vi "Fridge Software v2.1.vi"() -> ()   [LabVIEW 2017, in "Fridge Software v2.1.lvlib"]
uses:
  Fridge Software v2.1.lvlib
  <vilib>/Platform/TimedLoop/XDataNode/timing_clust.ctl
  <vilib>/Platform/TimedLoop/XDataNode/nitl_modes.ctl
  <vilib>/Platform/TimedLoop/XDataNode/wakeup.ctl
  <vilib>/Utility/file.llb/Write Delimited Spreadsheet (DBL).vi
  <vilib>/platform/TimedLoop/XDataNode/XDataNode.xnode
  <instrlib>/Lake Shore 372/Lake Shore 372.lvlib
  <instrlib>/Keithley 3706/Keithley 3700 Series.lvlib
  <vilib>/Platform/TimedLoop/XDataNode/XDNodeRunTimeDep.lvlib
panel:
  out "Input Reading Status Query":string
  out "Elapsed time":dbl=500.0 min=50.0 step=100.0
  out "Magnetic Poles \nLive  Voltage":dbl format="%#_5g"
  in  "Measurement\nperiod":i64=500 min=100 step=100
  out "Power Reading":dbl min=0.0 max=0.01 step=1e-05 format="%^.3g"
  out "Sample Reactance":dbl min=0.0 max=63200000.0 step=1e-05 format="%.3g"
  out "Cernox Resistance":dbl min=0.0 max=63200000.0 step=1e-05 format="%.3g"
  in  "R(T,H) tab":enum32{"R(T)", "R(H)"}(tab)
  in  "Clear R(T) graph":bool
  in  "Autoscale R(T)":bool=TRUE caption="Autoscale"
  out "R(T) Graph":cluster{dbl[], dbl[]}(graph)
  in  "Clear H(T) graph":bool
  in  "Autoscale H(T)":bool=TRUE caption="Autoscale"
  out "R(H) Graph":cluster{dbl[], dbl[]}(graph)
  in  "Clear H(t) graph":bool
  in  "Clear T(t) graph":bool
  in  "Clear R(t) graph":bool
  out "Sample Resistance":dbl min=0.0 max=63200000.0 step=1e-05 format="%^.5g"
  out "Cernox Temperature":dbl min=0.0 max=1000.0 step=1e-05 format="%.4f"
  in  "Autoscale H(t)":bool=TRUE caption="Autoscale"
  in  "Autoscale T(t)":bool=TRUE caption="Autoscale"
  in  "Autoscale R(t)":bool=TRUE caption="Autoscale"
  out "H(t) Graph 4":cluster{dbl[], dbl[]}(graph)
  out "T(t) Graph 3":cluster{dbl[], dbl[]}(graph)
  out "R(t) Graph":cluster{dbl[], dbl[]}(graph)
  in  "Measurement":T1(tab)
  in  "Hall probe/Aux":bool
  in  "Lakeshore port":refnum<visa-resource-name>="COM6"
  in  "Cernox Channel":u16(ring)=17 caption="Cernox" items=["1"=1, "2"=2, "3"=3, "4"=4, "5"=5, "6"=6, "7"=7, "8"=8, "9"=9, "10"=10, "11"=11, "12"=12, "13"=13, "14"=14, "15"=15, "16"=16, "A"=17]
  in  "Sample Channel":u16(ring)=1 caption="Sample" items=["1"=1, "2"=2, "3"=3, "4"=4, "5"=5, "6"=6, "7"=7, "8"=8, "9"=9, "10"=10, "11"=11, "12"=12, "13"=13, "14"=14, "15"=15, "16"=16, "A (Control Input)"=17]
  in  "Switchboard port":refnum<visa-resource-name>="USB0::0x05E6::0x3706::04089883::INSTR"
  in  "Arduino port \n(for magnetic poles)":refnum<visa-resource-name>="COM3"
  out "Lakeshore Error":errorcluster
  in  "Update":bool
  out "Excitation  Ind":bool=TRUE
  out "Excitation Mode Ind":u16(ring)=1 items=["Voltage", "Current"]
  out "Excitation Range Ind":u16(ring)=19 items=["31.6 mA"=22, "10.0 mA"=21, "3.16 mA"=20, "1.00 mA"=19, "316 uA"=18, "100 uA"=17, "31.6 uA"=16, "10.0 uA"=15, "3.16 uA"=14, "1.00 uA"=13, "632 mV / 316 nA"=12, "200 mV / 100 nA"=11, "63.2 mV / 31.6 nA"=10, "20.0 mV / 10.0 nA"=9, "6.32 mV / 3.16 nA"=8, "2.00 mV / 1.00 nA"=7, "632 uV / 316 pA"=6, "200 uV / 100 pA"=5, "63.2 uV / 31.6 pA"=4, "20.0 uV / 10.0 pA"=3, "6.32 uV / 3.16 pA"=2, "2.00 uV / 1.00 pA"=1]
  out "Autorange Ind":u16(ring) items=["Autorange off", "Autorange Current", "ROX 102B Autorange"]
  out "Resistance Range Ind":u16(ring)=8 items=["63.2 MOhm"=22, "20.0 MOhm"=21, "6.32 MOhm"=20, "2.00 MOhm"=19, "632 kOhm"=18, "200 kOhm"=17, "63.2 kOhm"=16, "20.0 kOhm"=15, "6.32 kOhm"=14, "2.00 kOhm"=13, "632 Ohm"=12, "200 Ohm"=11, "63.2 Ohm"=10, "20.0 Ohm"=9, "6.32 Ohm"=8, "2.00 Ohm"=7, "632 mOhm"=6, "200 mOhm"=5, "63.2 mOhm"=4, "20.0 mOhm"=3, "6.32 mOhm"=2, "2.00 mOhm"=1]
  out "Preferred Units Ind":u16(ring)=2 items=["Kelvin"=1, "Ohms"=2]
  out "Temperature Limit Ind":dbl min=0.0 max=2999.0 step=1.0
  in  "Excitation Mode":u16(ring)=1 items=["Voltage", "Current"]
  in  "Excitation Range":u16(ring)=19 items=["31.6 mA"=22, "10.0 mA"=21, "3.16 mA"=20, "1.00 mA"=19, "316 uA"=18, "100 uA"=17, "31.6 uA"=16, "10.0 uA"=15, "3.16 uA"=14, "1.00 uA"=13, "632 mV / 316 nA"=12, "200 mV / 100 nA"=11, "63.2 mV / 31.6 nA"=10, "20.0 mV / 10.0 nA"=9, "6.32 mV / 3.16 nA"=8, "2.00 mV / 1.00 nA"=7, "632 uV / 316 pA"=6, "200 uV / 100 pA"=5, "63.2 uV / 31.6 pA"=4, "20.0 uV / 10.0 pA"=3, "6.32 uV / 3.16 pA"=2, "2.00 uV / 1.00 pA"=1]
  in  "Autorange (0: Autorange off)":u16(ring) items=["Autorange off", "Autorange Current", "ROX 102B Autorange"]
  in  "Resistance Range":u16(ring)=8 items=["63.2 MOhm"=22, "20.0 MOhm"=21, "6.32 MOhm"=20, "2.00 MOhm"=19, "632 kOhm"=18, "200 kOhm"=17, "63.2 kOhm"=16, "20.0 kOhm"=15, "6.32 kOhm"=14, "2.00 kOhm"=13, "632 Ohm"=12, "200 Ohm"=11, "63.2 Ohm"=10, "20.0 Ohm"=9, "6.32 Ohm"=8, "2.00 Ohm"=7, "632 mOhm"=6, "200 mOhm"=5, "63.2 mOhm"=4, "20.0 mOhm"=3, "6.32 mOhm"=2, "2.00 mOhm"=1]
  in  "Preferred Units (2: Ohms)":u16(ring)=2 items=["Kelvin"=1, "Ohms"=2]
  in  "Temperature Limit (0 Kelvin)":dbl min=0.0 max=2999.0 step=1.0
  in  "Excitation  (T: On)":bool=TRUE caption="On\n\nOff"
  in  "Grab settings":bool
  out "Heater Output Ind":dbl
  in  "Heater Setpoint":dbl
  out "Heater Setpoint Ind":dbl
  in  "Grab Heater settings":bool
  in  "Update Heater Settings":bool
  in  "Excitation  (T: On) 2":bool=TRUE caption="On\n\nOff"
  out "Excitation  Ind 2":bool=TRUE
  out "Heater Output Ind 2":dbl
  in  "I+":i32 min=0 max=24 step=1
  in  "I-":i32 min=0 max=24 step=1
  in  "V+":i32 min=0 max=24 step=1
  in  "V-":i32 min=0 max=24 step=1
  in  "Close pins (safe)":bool caption="Close I-V pins -> Lift ground -> Lift common -> Current on"
  in  "Lift pins (safe)":bool caption="Current off -> Common closed -> Ground -> Lift I-V pins"
  in  "Channel Open/Close Array":string
  in  "Open":bool
  in  "Close":bool
  in  "Open All IV":bool
  out "Closed Channels":string
  out "Ground closed":bool
  out "Common rail \nclosed":bool
  out "Common-ground \nlink closed":bool
  in  "Append file":bool
  in  "File path":path
  in  "Save Data":bool
  in  "error in":errorcluster
  in  "Aux max voltage (mV)":dbl
  in  "Aux Field Range (Oe)":dbl
  in  "Stop":bool
  # "Created by Daniel Bromley & Alex Wright, IPF Ltd 2021"
  # "s"
  # "V"
  # "ms"
  # "W"
  # "jW"
  # "W"
  # "W"
  # "K"
  # "Lakeshore - Measurement"
  # "Channels:"
  # "Keithley - Switchboard"
  # "Hall probe"
  # "Aux"
  # "Excitation Mode"
  # "Excitation Range"
  # "Autorange"
  # "Resistance Range"
  # "Preferred Units"
  # "Temperature Limit"
  # "Excitation"
  # "Heater Serpoint (K)"
  # "Heater output"
  # "Heater On"
  # "IV pins"
  # "Array"
  # "Set Filename and Path"
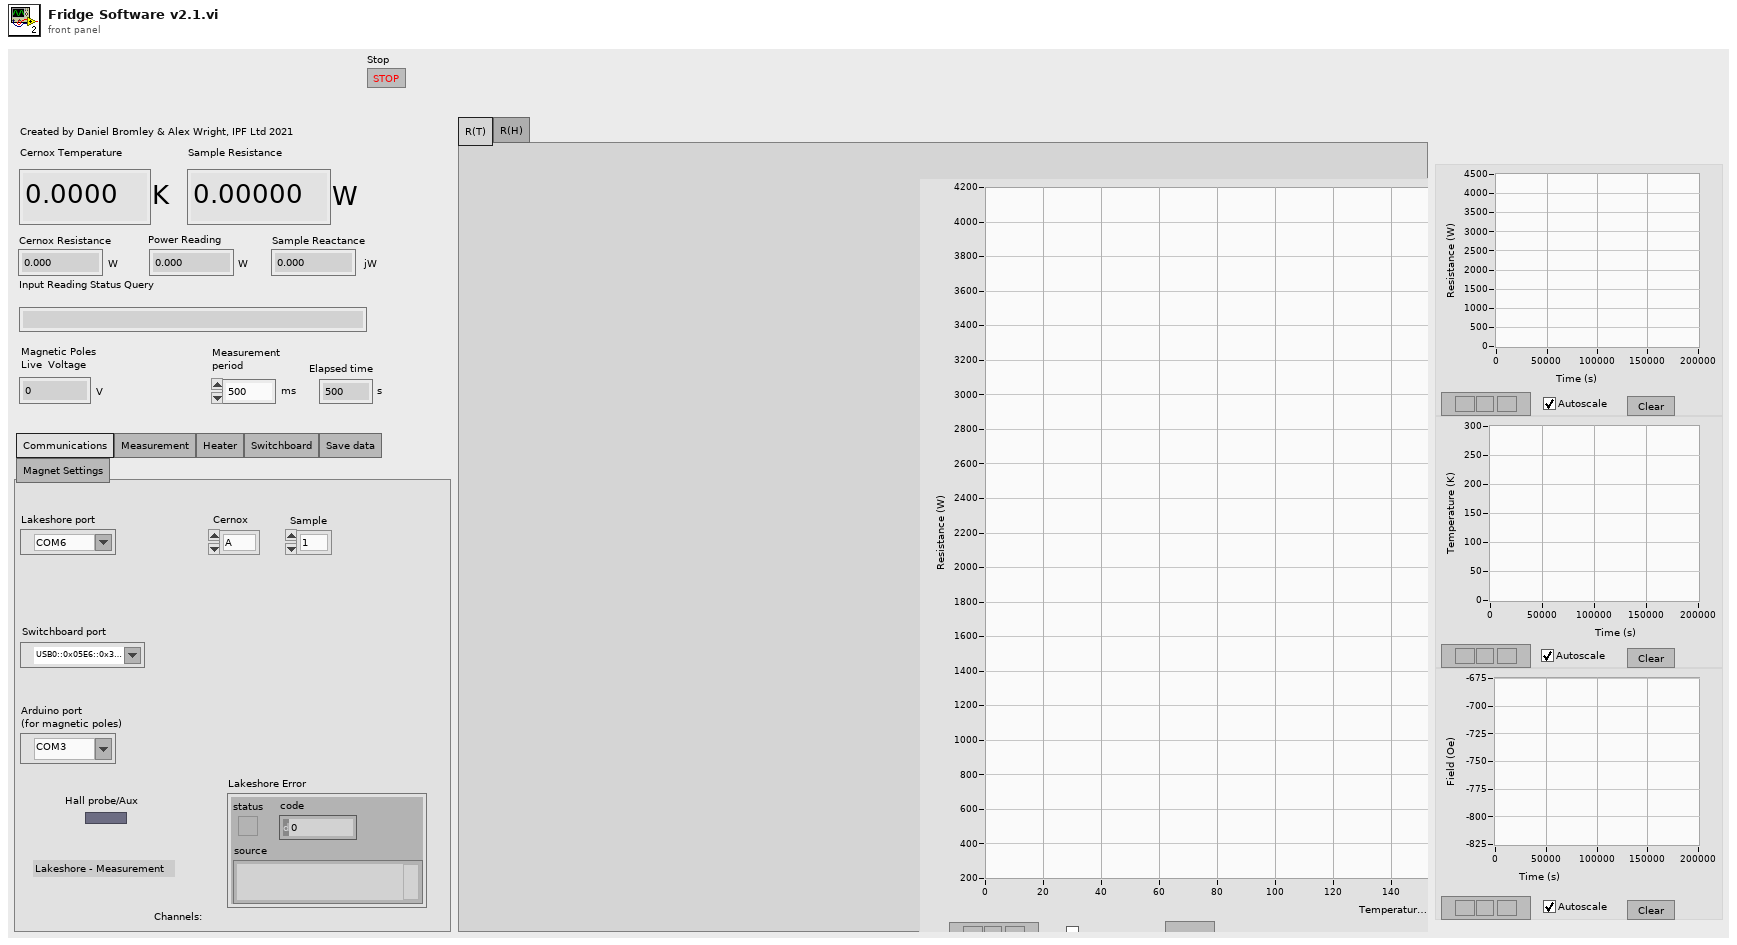
[diagram p1: front panel]
types:
  T1 = enum32{"Communications", "Measurement", "Heater", "Switchboard", "Save data", "Magnet Settings"}
  T2 = typedef "XDNodeRunTimeDep.lvlib/timing_clust.ctl" = cluster{"Expected End [f-1]":u64, "Actual End [f-1]":u64, "Finished Late? [f-1]":bool, "Expected End [i-1]":u64, "Actual End [i-1]":u64, "Finished Late? [i-1]":bool, "Expected Start [i]":u64, "Actual Start [i]":u64, "Expected Start [f]":u64, "Actual Start [f]":u64, "Source Name":string, "Structure Name":string, "Period":i64, "Deadline":i64, "Offset":i64, "Start":i64, "Priority":i32, "Timeout":i32, "Mode":T3, "Wakeup Reason":T4, "Error":errorcluster, "Source Type":string, "Secondary Source Type":string, "Global End Time":u64, "Global Start Time":u64, "Frame Duration":u64, "Iteration Duration":u64, "Assigned CPU":i32, "I/O Scan Engine Mode":u32}
  T3 = typedef "XDNodeRunTimeDep.lvlib/nitl_modes.ctl" = enum32{"No Change", "Process missed periods, maintain original phase", "Discard missed periods, maintain original phase", "Process missed periods, ignore original phase", "Discard missed periods, ignore original phase"}
  T4 = typedef "XDNodeRunTimeDep.lvlib/wakeup.ctl" = enum32{"Normal", "Aborted", "Asynchronous wakeup", "Timing source error", "Timed loop error", "Timeout"}
  T5 = typedef "eventsource.ctl" = u32
  T6 = typedef "lveventtype.ctl" = enum32{"Null", "Timeout", "Annotation Menu Selection", "Annotation Menu Selection?", "App Instance Close", "App Instance Close?", "Autoscale Range Change", "Bookmark Info Change", "Cell Edit", "Cell Edit?", "Cursor Grab", "Cursor Grab?", "Cursor Menu Selection", "Cursor Menu Selection?", "Cursor Move", "Cursor Release", "Data Change", "Direction Change", "Display State Change", "Drag Ended", "Drag Enter", "Drag Leave", "Drag Over", "Drag Source Update", "Drag Starting", "Drag Starting?", "Drop", "Exec State Change", "Key Down", "Key Down?", "Key Repeat", "Key Repeat?", "Key Up", "Listbox Double Click", "Menu Activation?", "Menu Selection (App)", "Menu Selection? (App)", "Menu Selection (User)", "Mouse Down", "Mouse Down?", "Mouse Enter", "Mouse Leave", "Mouse Move", "Mouse Up", "Mouse Wheel", "NI Security User Change (App)", "Pane Size", "Panel Close", "Panel Close?", "Panel Resize", "Plot Attribute Change", "Scale Range Change", "Shortcut Menu Activation?", "Shortcut Menu Selection (App)", "Shortcut Menu Selection? (App)", "Shortcut Menu Selection (User)", "Tree Double Click", "Tree Drag", "Tree Drag?", "Tree Drop", "Tree Drop?", "Tree Item Close", "Tree Item Close?", "Tree Item Open", "Tree Item Open?", "User Event", "Value Change"}
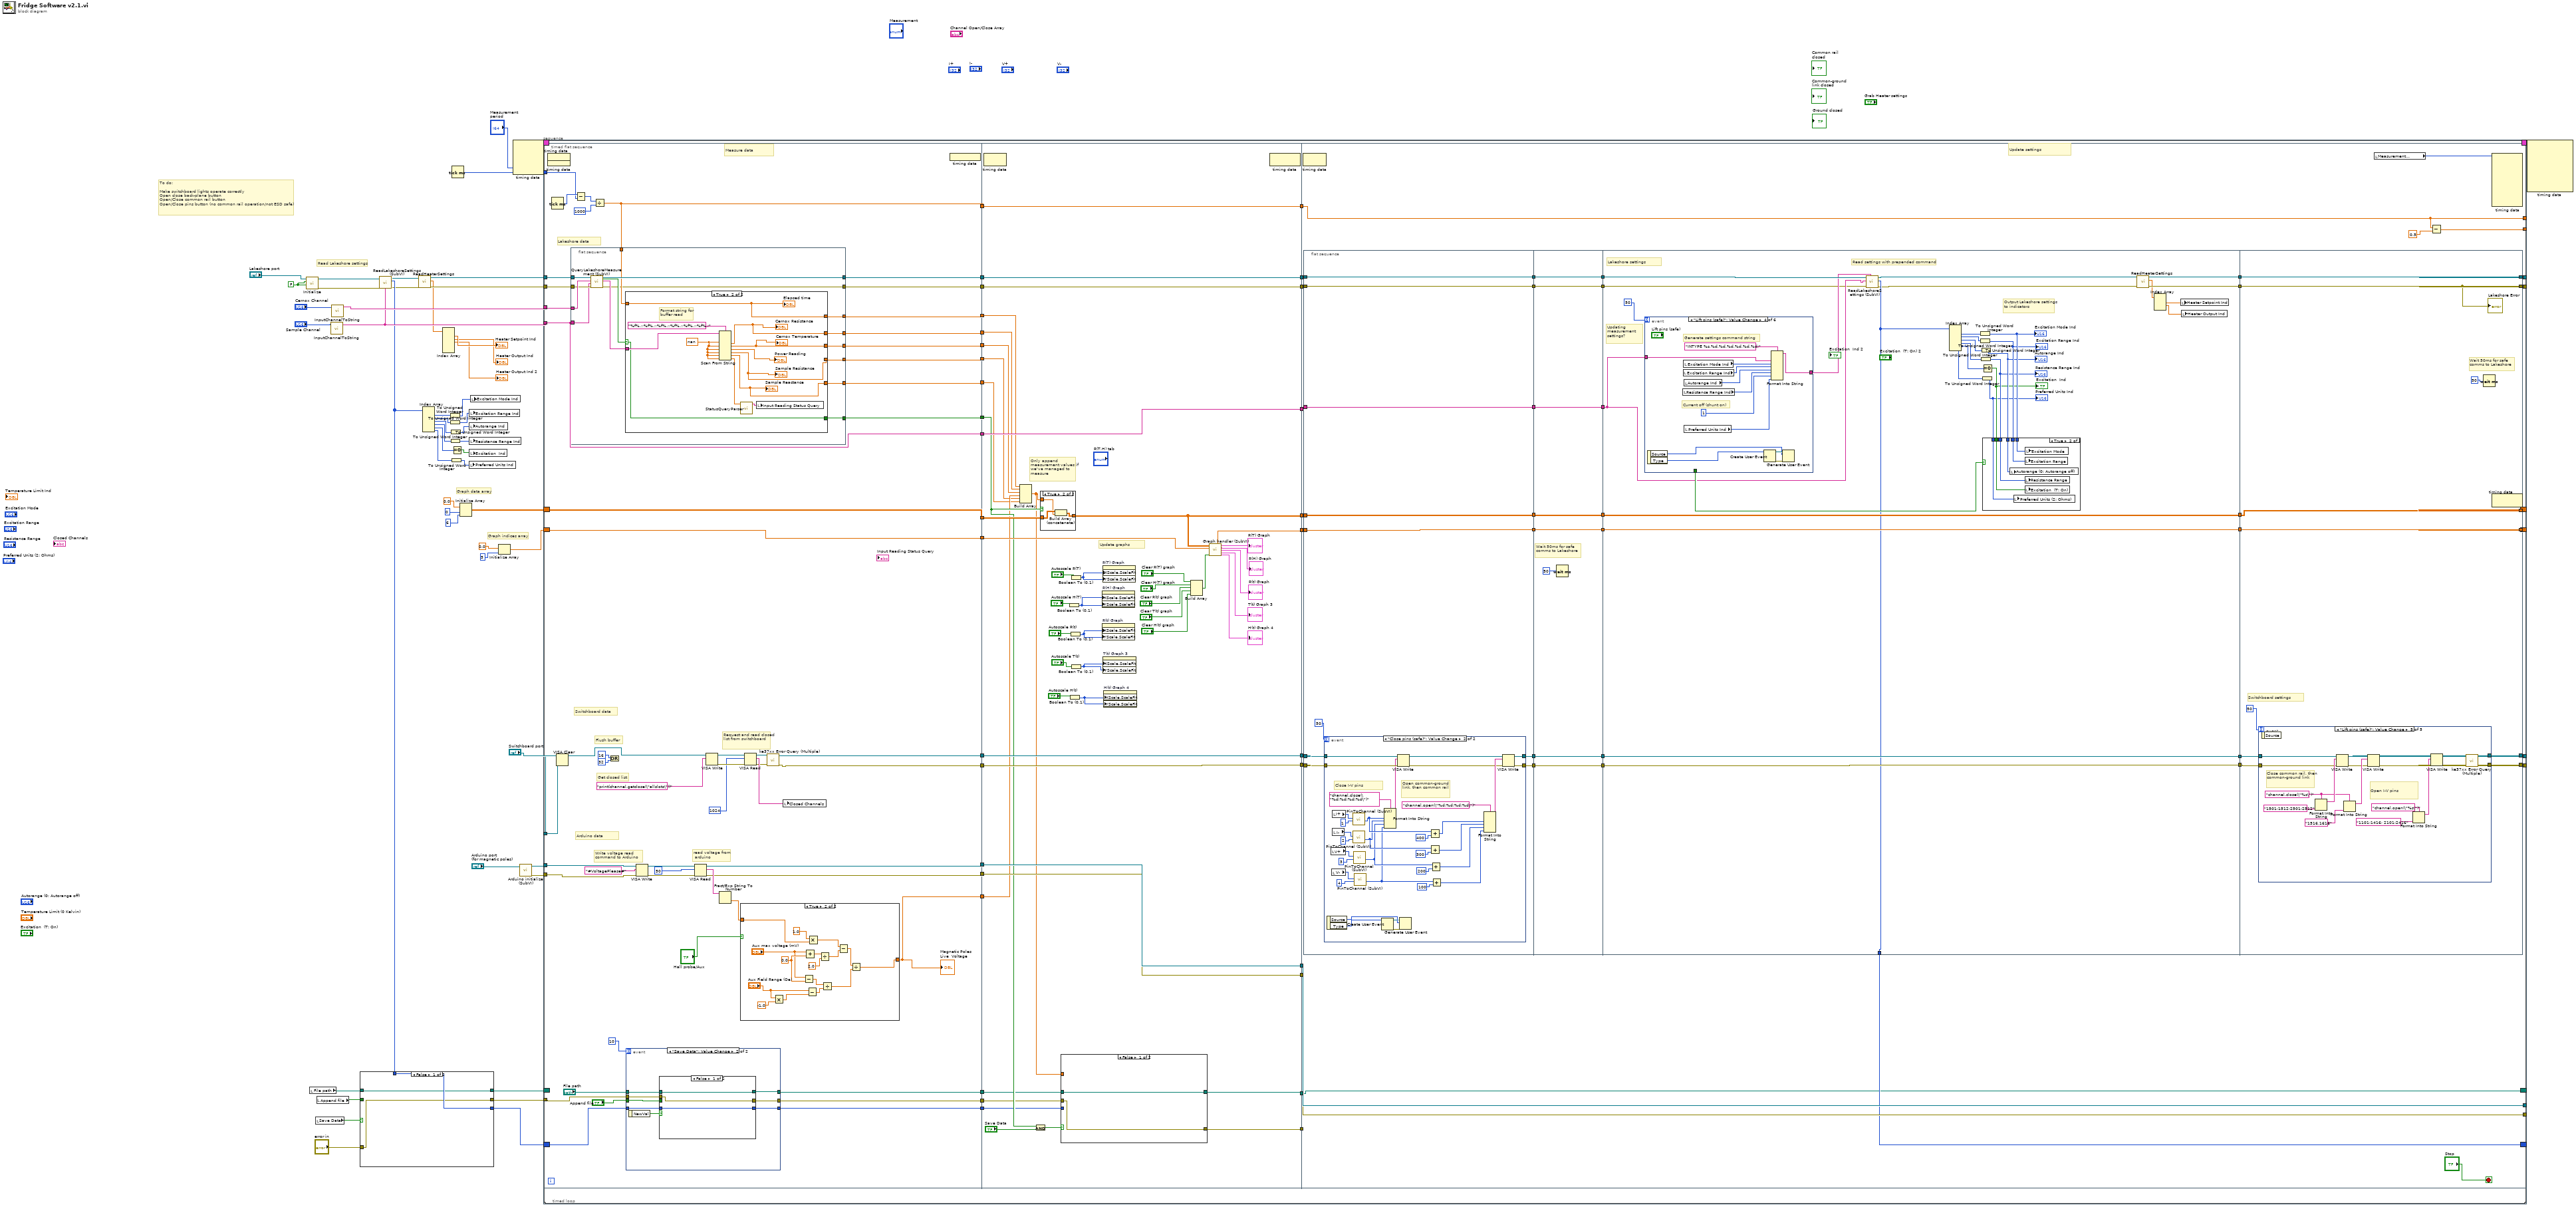
[diagram p0: block diagram]
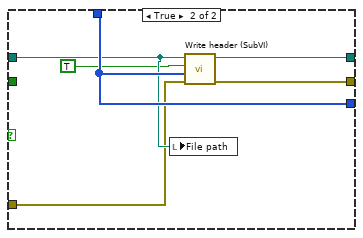
[diagram p2: hidden frame]
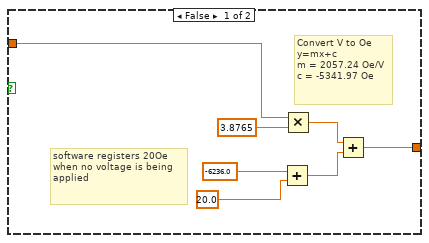
[diagram p3: hidden frame]
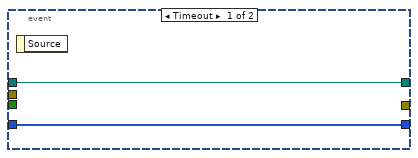
[diagram p4: hidden frame]
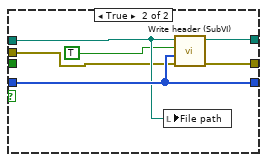
[diagram p5: hidden frame]
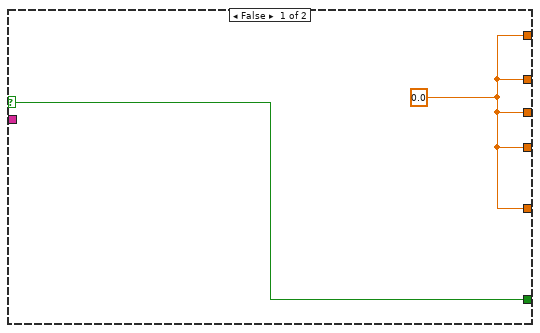
[diagram p6: hidden frame]
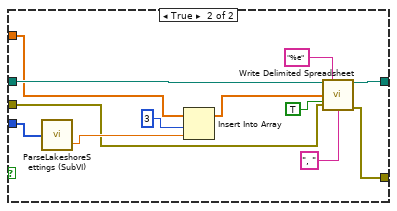
[diagram p7: hidden frame]
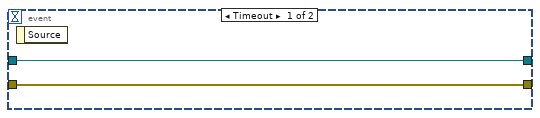
[diagram p9: hidden frame]
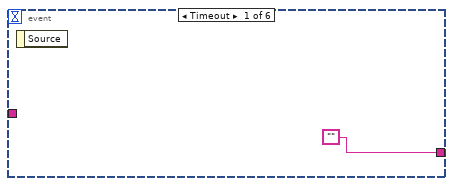
[diagram p10: hidden frame]
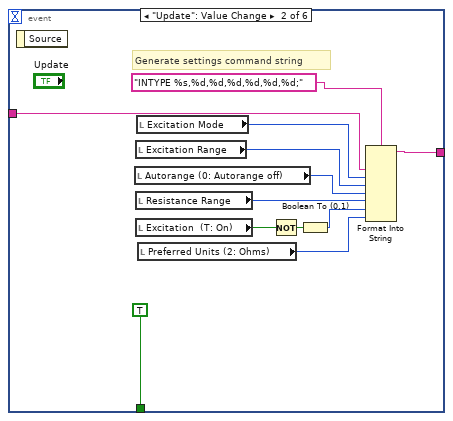
[diagram p11: hidden frame]
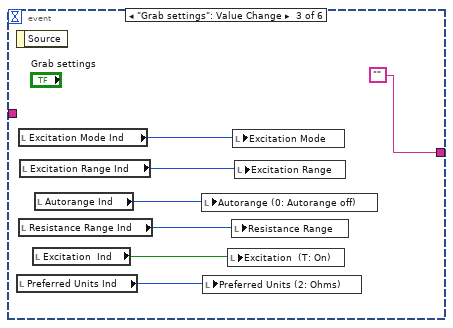
[diagram p12: hidden frame]
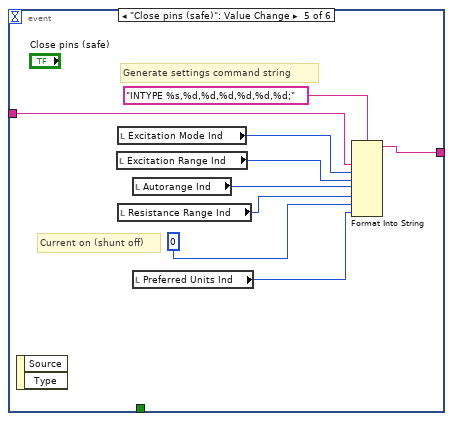
[diagram p13: hidden frame]
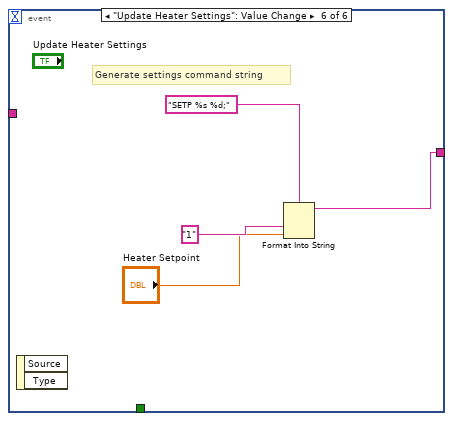
[diagram p14: hidden frame]
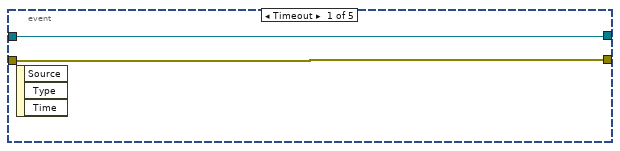
[diagram p16: hidden frame]
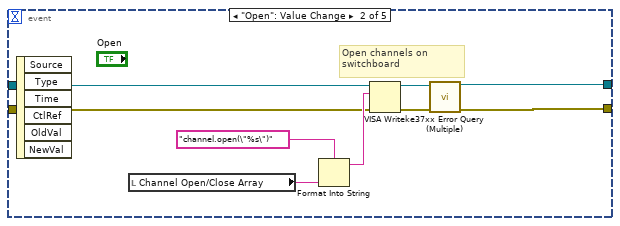
[diagram p17: hidden frame]
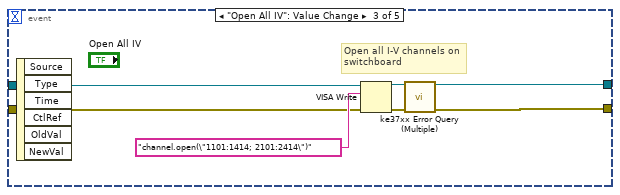
[diagram p18: hidden frame]
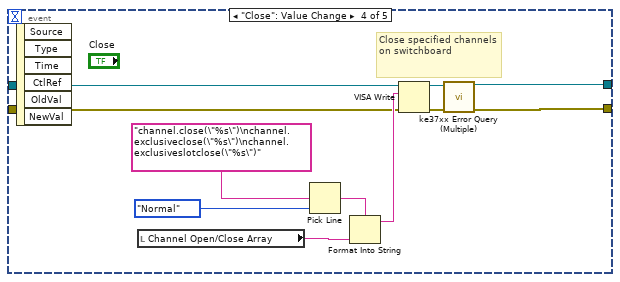
[diagram p19: hidden frame]
diagram:
  w12 = FALSE
  # "To do:\n\nMake switchboard lights operate correctly\nOpen close back-plane button\nOpen/Close common rail button\nOpen/Close pins button (no common rail operation/not ESD safe)"
  # "Read Lakeshore settings"
  # "Graph indices array"
  # "Graph data array"
  n1 = call <instrlib>:"Initialize.vi"("Reset (True)"=w12, "ID Query (True)"=w12, "VISA resource name"="Lakeshore port") -> ("error out"=w11:errorcluster, "VISA resource name out"=w32:refnum<visa-resource-name>)  [unwired: 7 in]
  n2 = local read "File path"() -> (w13:path)
  n3 = local read "Save Data"() -> (w24:bool)
  n4 = local read "Append file"() -> (w23:bool)
  n5 = call <instrlib>:"InputChannelToString.vi"("Channel (1)"="Sample Channel") -> ("Channel Str"=w28:string)  [unwired: 10 in]
  n6 = call <instrlib>:"InputChannelToString.vi"("Channel (1)"="Cernox Channel") -> ("Channel Str"=w30:string)  [unwired: 10 in]
  n7 = call "ReadLakeshoreSettings (SubVI).vi"("error in (no error)"=w11, "Channel Str"=w28, "Lakeshore port"=w32) -> ("error out"=w8:errorcluster, "Settings array out"=w22:i32[], "VISA Refnum out"=w10:refnum<visa-resource-name>)  [unwired: 4 in]
  n8 = case shown="False" w24 {
    tunnel: w23 -> [_ _]
    tunnel: w22 -> [w55 w61]
    tunnel: [w55 w61] -> w21
    tunnel: [w54 w60] -> w14
    tunnel: w13 -> [w54 w59]
    tunnel: [w53 w57] -> w2
    tunnel: "error in" -> [w53 w56]
    frame False {
    }
    frame True {
      n9 = local write "File path"(w59) -> ()
      n10 = call "Write header (SubVI).vi"("error in"=w56, "Settings array in"=w61, "Append? Out"=TRUE, "Path in"=w59) -> ("error out"=w57:errorcluster, "Path out"=w60:path)  [unwired: 6 in]
    }
  }
  n11 = call "ReadHeaterSettings.vi"("error in (no error)"=w8, "VISA Refnum in"=w10) -> ("error out"=w7:errorcluster, "Settings array out"=w6:dbl[], "VISA Refnum out"=w9:refnum<visa-resource-name>)  [unwired: 7 in]
  n12 = Index Array(array=w22) -> (element #1=w38:i32, element #2=w37:i32, element #3=w36:i32, element #4=w35:i32, element #5=w34:i32, element #6=w33:i32)  [unwired: 6 in]
  n13 = Index Array(array=w6) -> (element #1=→"Heater Setpoint Ind":dbl, element #2=→"Heater Output Ind":dbl, element #3=→"Heater Output Ind 2":dbl)  [unwired: 6 in, 3 out]
  n14 = To Unsigned Word Integer(number=w38) -> (unsigned 16bit integer=w20:u16)
  n15 = To Unsigned Word Integer(number=w37) -> (unsigned 16bit integer=w19:u16)
  n16 = To Unsigned Word Integer(number=w35) -> (unsigned 16bit integer=w17:u16)
  n17 = To Unsigned Word Integer(number=w36) -> (unsigned 16bit integer=w18:u16)
  n18 = To Unsigned Word Integer(number=w33) -> (unsigned 16bit integer=w15:u16)
  n19 = Equal To 0?(x=w34) -> (x = 0?=w16:bool)
  n20 = Tick Count (ms)() -> (millisecond timer value=w51:u32)
  n21 = Initialize Array(0.0, 0, 6) -> (w42:dbl[][])
  n22 = local write "Preferred Units Ind"(w15) -> ()
  n23 = local write "Excitation Range Ind"(w19) -> ()
  n24 = local write "Autorange Ind"(w18) -> ()
  n25 = local write "Resistance Range Ind"(w17) -> ()
  n26 = local write "Excitation  Ind"(w16) -> ()
  n27 = local write "Excitation Mode Ind"(w20) -> ()
  n28 = Initialize Array(0.0, 5) -> (w39:dbl[])
  n29 = node-c288("Measurement\nperiod") -> (w50:T2)  [unwired: 3 in]
  n30 = call "Arduino initialize (SubVI).vi"("VISA Refnum in"="Arduino port \n(for magnetic poles)") -> ("error out"=w25:errorcluster, "VISA Refnum out"=w26:refnum<visa-resource-name>)  [unwired: 9 in]
  n31 = VISA Clear(VISA resource name="Switchboard port") -> (VISA resource name out=w46:refnum<visa-resource-name>)  [unwired: 1 in, 1 out]
  n32 = timed-loop {
    timing: w50 -> [_]
    timing-out: [_] -> w49
    tunnel: w30 -> [w86]
    tunnel: w28 -> [w85]
    tunnel: w7 -> [w84]
    tunnel: w9 -> [w83]
    tunnel: w26 -> [w82]
    tunnel: w25 -> [w81]
    tunnel: [w80] -> _
    tunnel: [w79] -> _
    tunnel: [w78] -> _
    tunnel: [w77] -> _
    tunnel: w46 -> [w76]
    tunnel: w51 -> [w75]
    tunnel: [w74] -> _
    tunnel: [w73] -> _
    shift-right: [w72] -> _
    shift-left: w42 -> [w71]
    shift-right: [w70] -> _
    shift-left: w39 -> [w69]
    tunnel: [w68] -> _
    tunnel: [w67] -> _
    shift-right: [w66] -> _
    shift-left: w21 -> [w65]
    shift-right: [w64] -> _
    shift-left: w14 -> [w63]
    tunnel: w2 -> [w62]
    stop <- "Stop" stop-if-true
    n33 = timed-sequence {
      timing: _ -> [_]
      timing-out: _ -> [_]
      tunnel: w86 -> [w140]
      tunnel: w85 -> [w143]
      tunnel: w84 -> [w142]
      tunnel: w83 -> [w141]
      tunnel: w82 -> [w135]
      tunnel: w81 -> [w134]
      tunnel: [w139] -> w80
      tunnel: [w138] -> w79
      tunnel: [w137] -> w78
      tunnel: [w136] -> w77
      tunnel: w76 -> [w133]
      tunnel: w75 -> [w132]
      tunnel: [w131] -> w74
      tunnel: [w130] -> w73
      tunnel: [w129] -> w72
      tunnel: w71 -> [w128]
      tunnel: [w102] -> w70
      tunnel: w69 -> [w100]
      tunnel: [w98] -> w68
      tunnel: [w97] -> w67
      tunnel: [w96] -> w66
      tunnel: w65 -> [w95]
      tunnel: [w94] -> w64
      tunnel: w63 -> [w93]
      tunnel: w62 -> [w89]
      n34 = timed-flat-sequence {
        tunnel: w143 -> [w192]
        tunnel: [w194] -> w127
        tunnel: [w193] -> w125
        tunnel: [w192] -> w123
        tunnel: w142 -> [w191]
        tunnel: w141 -> [w190]
        tunnel: w140 -> [w189]
        tunnel: [w185] -> w121
        tunnel: [w184] -> w119
        tunnel: w135 -> [w170]
        tunnel: w134 -> [w169]
        tunnel: w133 -> [w171]
        tunnel: [w156] -> w117
        tunnel: [w155] -> w115
        tunnel: w132 -> [w167]
        tunnel: [w158] -> w113
        tunnel: w128 -> [w166]
        tunnel: [w166] -> w111
        tunnel: [w165] -> w110
        tunnel: [w164] -> w109
        tunnel: [w163] -> w108
        tunnel: [w162] -> w107
        tunnel: [w161] -> w106
        tunnel: [w146] -> w105
        tunnel: [w160] -> w103
        tunnel: [w159] -> w101
        tunnel: w100 -> [w159]
        tunnel: w95 -> [w154]
        tunnel: w93 -> [_]
        tunnel: [w150] -> w92
        tunnel: [w149] -> w90
        tunnel: w89 -> [w145]
        tunnel: [w144] -> w88
        tunnel: w127 -> [w315]
        tunnel: [w315] -> w126
        tunnel: w125 -> [w314]
        tunnel: [w314] -> w124
        tunnel: w123 -> [w313]
        tunnel: [w313] -> w122
        tunnel: w121 -> [w312]
        tunnel: [w312] -> w120
        tunnel: w119 -> [w311]
        tunnel: [w311] -> w118
        tunnel: w117 -> [w310]
        tunnel: [w310] -> w116
        tunnel: w115 -> [w309]
        tunnel: [w309] -> w114
        tunnel: w113 -> [w308]
        tunnel: [w308] -> w112
        tunnel: w111 -> [w307]
        tunnel: w110 -> [w306]
        tunnel: w109 -> [w305]
        tunnel: w108 -> [w304]
        tunnel: w107 -> [w271]
        tunnel: w106 -> [w270]
        tunnel: w105 -> [w272]
        tunnel: [w288] -> w104
        tunnel: w103 -> [w278]
        tunnel: w101 -> [w287]
        tunnel: [w285] -> w99
        tunnel: w92 -> [w275]
        tunnel: [w274] -> w91
        tunnel: w90 -> [w273]
        tunnel: w88 -> [w269]
        tunnel: [w268] -> w87
        tunnel: w126 -> [w377]
        tunnel: w124 -> [w376]
        tunnel: w122 -> [w375]
        tunnel: [w374] -> w139
        tunnel: [w373] -> w138
        tunnel: w120 -> [w372]
        tunnel: w118 -> [w371]
        tunnel: [w372] -> w137
        tunnel: [w371] -> w136
        tunnel: w116 -> [w366]
        tunnel: w114 -> [w365]
        tunnel: w112 -> [w339]
        tunnel: [w368] -> w131
        tunnel: [w367] -> w130
        tunnel: [w346] -> w129
        tunnel: w104 -> [w348]
        tunnel: [w341] -> w102
        tunnel: w99 -> [w344]
        tunnel: [w339] -> w98
        tunnel: [w338] -> w97
        tunnel: [w337] -> w96
        tunnel: [w336] -> w94
        tunnel: w91 -> [w336]
        tunnel: w87 -> [_]
        frame #0 {
          # "Request and read closed list from switchboard"
          # "Get closed list"
          # "Flush buffer"
          # "Switchboard data"
          # "Arduino data"
          # "Lakeshore data"
          # "read voltage from\n arduino"
          # "Write voltage read command to Arduino"
          # "Measure data"
          n35 = node-c288() -> ()  [unwired: 1 in]
          n36 = Tick Count (ms)() -> (millisecond timer value=w168:u32)
          n37 = flat-sequence {
            tunnel: w192 -> [w245]
            tunnel: w191 -> [w249]
            tunnel: w190 -> [w248]
            tunnel: w189 -> [w250]
            tunnel: [w251] -> w194
            tunnel: [w237] -> w193
            tunnel: w158 -> [w244]
            tunnel: [w243] -> w165
            tunnel: [w242] -> w164
            tunnel: [w241] -> w163
            tunnel: [w240] -> w162
            tunnel: [w239] -> w161
            tunnel: [w238] -> w160
            frame #0 {
              n38 = call "QueryLakeshoreMeasurement (SubVI).vi"("error in (no error)"=w249, "Sample Channel Str"=w245, "Cernox channel string"=w250, "VISA Refnum in"=w248) -> ("error out"=w237:errorcluster, "Read output"=w247:string, "VISA Refnum out"=w251:refnum<visa-resource-name>, "Boolean"=w246:bool)  [unwired: 4 in]
              n39 = case shown="True" w246 {
                selector: w246 -> [w252 w262]
                tunnel: w247 -> [_ w264]
                tunnel: w244 -> [_ w259]
                tunnel: [w253 w259] -> w243
                tunnel: [w253 w257] -> w242
                tunnel: [w253 w256] -> w241
                tunnel: [w253 w254] -> w240
                tunnel: [w253 w258] -> w239
                tunnel: [w252 w262] -> w238
                frame False {
                  w253 = 0.0
                }
                frame True {
                  w263 = nan
                  # "Format string for buffer read"
                  n40 = Scan From String(format string="%f%.;;%f%.;;%f%.;;%f%.;;%f%.;;%f%.;", input string=w264, default 1=w263, default 2=w263, default 3=w263, default 4=w263, default 5=w263, default 6=w263) -> (output 1=w257:dbl, output 2=w256:dbl, output 3=→"Power Reading":dbl, output 4=w254:dbl, output 5=w258:dbl, output 6=w261:dbl)  [unwired: 2 in, 3 out]
                  "Sample Reactance" <- w258
                  "Cernox Resistance" <- w257
                  "Cernox Temperature" <- w256
                  "Sample Resistance" <- w254
                  n41 = call "StatusQueryParser.vi"("Numeric"=w261) -> ("String"=w260:string)  [unwired: 10 in]
                  n42 = local write "Input Reading Status Query"(w260) -> ()
                  "Elapsed time" <- w259
                }
              }
            }
          }
          n43 = Subtract(x=w168, y=w167) -> (x-y=w174:u32)
          n44 = Divide(x=w174, y=1000) -> (x/y=w158:dbl)
          n45 = Or(x=16, y=32) -> ()  [unwired: 1 out]
          n46 = event shown="[1] \"Save Data\": Value Change" {
            selector: _ -> [_ _]
            dyn-events: _ -> [_ _]
            timeout: 10 -> [_ _]
            tunnel: w154 -> [w218 w226]
            tunnel: "Append file" -> [_ w225]
            tunnel: "File path" -> [w219 w224]
            tunnel: [w219 w223] -> w150
            tunnel: [w218 w222] -> w149
            tunnel: w145 -> [_ w221]
            tunnel: [_ w220] -> w144
            event Timeout {
              n47 = event-data() -> ()  [unwired: 1 in, 1 out]
            }
            event "Save Data": Value Change {
              n48 = event-data() -> ("NewVal"=w227:bool)  [unwired: 1 in]
              n49 = case shown="False" w227 {
                tunnel: w226 -> [w229 w235]
                tunnel: w225 -> [_ _]
                tunnel: w224 -> [w230 w234]
                tunnel: [w230 w236] -> w223
                tunnel: [w229 w235] -> w222
                tunnel: w221 -> [w228 w232]
                tunnel: [w228 w231] -> w220
                frame False {
                }
                frame True {
                  n50 = local write "File path"(w234) -> ()
                  n51 = call "Write header (SubVI).vi"("error in"=w232, "Settings array in"=w235, "Append? Out"=TRUE, "Path in"=w234) -> ("error out"=w231:errorcluster, "Path out"=w236:path)  [unwired: 6 in]
                }
              }
            }
          }
          n52 = VISA Write(VISA resource name=w170, write buffer="#VoltagePlease#" ("Send to Arduino"), error in (no error)=w169) -> (VISA resource name out=w186:refnum<visa-resource-name>, error out=w183:errorcluster)  [unwired: 1 out]
          n53 = VISA Read(VISA resource name=w186, byte count=u32 50 ("milliseconds to wait"), error in (no error)=w183) -> (VISA resource name out=w185:refnum<visa-resource-name>, read buffer=w188:string, error out=w184:errorcluster)  [unwired: 1 out]
          n54 = VISA Write(VISA resource name=w171, write buffer="print(channel.getclose(\"allslots\"))") -> (VISA resource name out=w180:refnum<visa-resource-name>, error out=w179:errorcluster)  [unwired: 1 in, 1 out]
          n55 = Fract/Exp String To Number(string=w188) -> (number=w147:dbl)  [unwired: 3 in, 1 out]
          n56 = case shown="True" "Hall probe/Aux" {
            tunnel: w147 -> [w196 w209]
            tunnel: [w195 w206] -> w146
            frame False {
              # "software registers 20Oe when no voltage is being applied"
              # "Convert V to Oe\ny=mx+c\nm = 2057.24 Oe/V\nc = -5341.97 Oe"
              n57 = Add(x=-6236.0, y=20.0) -> (x+y=w200:dbl)
              n58 = Multiply(x=w196, y=3.8765) -> (x*y=w201:dbl)
              n59 = Add(x=w201, y=w200) -> (x+y=w195:dbl)
            }
            frame True {
              w214 = 0.0
              n60 = Multiply(x="Aux Field Range (Oe)", y=-1.0) -> (x*y=w204:dbl)
              n61 = Subtract(x="Aux max voltage (mV)", y=w214) -> (x-y=w213:dbl)
              n62 = Add(x="Aux max voltage (mV)", y=w214) -> (x+y=w217:dbl)
              n63 = Subtract(x="Aux Field Range (Oe)", y=w204) -> (x-y=w212:dbl)
              n64 = Multiply(x=1.0, y=w209) -> (x*y=w207:dbl)
              n65 = Divide(x=w217, y=2.0) -> (x/y=w215:dbl)
              n66 = Divide(x=w213, y=w212) -> (x/y=w210:dbl)
              n67 = Subtract(x=w207, y=w215) -> (x-y=w211:dbl)
              n68 = Divide(x=w211, y=w210) -> (x/y=w206:dbl)
            }
          }
          "Magnetic Poles \nLive  Voltage" <- w146
          n69 = VISA Read(VISA resource name=w180, byte count=u32 1024 ("Bytes To Read (1024)"), error in (no error)=w179) -> (VISA resource name out=w181:refnum<visa-resource-name>, read buffer=w172:string, error out=w157:errorcluster)  [unwired: 1 out]
          n70 = call <instrlib>:"ke37xx Error Query (Multiple).vi"("VISA resource name"=w181, "error in (no error)"=w157) -> ("VISA resource name out"=w156:refnum<visa-resource-name>, "error out"=w155:errorcluster)  [unwired: 10 in, 2 out]
          n71 = local write "Closed Channels"(w172) -> ()
          n72 = node-c288() -> ()  [unwired: 1 out]
        }
        frame #1 {
          # "Update graphs"
          # "Only append measurement values if we've managed to measure"
          n73 = node-c288() -> ()  [unwired: 1 in, 1 out]
          n74 = Build Array(w306, w305, w304, w272, w271, w270) -> (w276:dbl[])
          n75 = And(x=w278, y="Save Data") -> (x .and. y?=w277:bool)
          n76 = case shown="True" w278 {
            tunnel: w307 -> [w330 w332]
            tunnel: w276 -> [_ w331]
            tunnel: [w330 w333] -> w288
            frame False {
            }
            frame True {
              n77 = Build Array (concatenate)(w332, w331) -> (w333:dbl[][])
            }
          }
          n78 = case shown="False" w277 {
            tunnel: w276 -> [_ w323]
            tunnel: w275 -> [w317 w329]
            tunnel: [w317 w328] -> w274
            tunnel: w273 -> [_ w321]
            tunnel: w269 -> [w316 w319]
            tunnel: [w316 w318] -> w268
            frame False {
            }
            frame True {
              n79 = call "ParseLakeshoreSettings (SubVI).vi"("Settings array in"=w321) -> ("Current excitation (A)"=w320:dbl)  [unwired: 1 out]
              n80 = Insert Into Array(array=w323, index=3, new element=w320) -> (w322:dbl[])
              n81 = call-poly <vilib>:"Write Delimited Spreadsheet.vi"("file path (dialog if empty)"=w329, "format (%.3f)"="%e", "1D data"=w322, "append to file? (new file:F)"=TRUE, "error in (no error)"=w319, "delimiter (\\t)"=", ") -> ("new file path (Not A Path if cancelled)"=w328:path, "error out"=w318:errorcluster)  [unwired: 8 in]
            }
          }
          n82 = Boolean To (0,1)(Boolean="Autoscale H(T)") -> (0, 1=w289:i16)
          n83 = Boolean To (0,1)(Boolean="Autoscale H(t)") -> (0, 1=w296:i16)
          n84 = Boolean To (0,1)(Boolean="Autoscale R(t)") -> (0, 1=w300:i16)
          n85 = Boolean To (0,1)(Boolean="Autoscale R(T)") -> (0, 1=w302:i16)
          n86 = Boolean To (0,1)(Boolean="Autoscale T(t)") -> (0, 1=w298:i16)
          n87 = property on="R(H) Graph" class="XYGraph (strict)"("XScale.ScaleFit"=w289, "YScale.ScaleFit"=w289) -> ()  [unwired: 2 in, 2 out]
          n88 = property on="R(t) Graph" class="XYGraph (strict)"("XScale.ScaleFit"=w300, "YScale.ScaleFit"=w300) -> ()  [unwired: 2 in, 2 out]
          n89 = property on="R(T) Graph" class="XYGraph (strict)"("XScale.ScaleFit"=w302, "YScale.ScaleFit"=w302) -> ()  [unwired: 2 in, 2 out]
          n90 = property on="T(t) Graph 3" class="XYGraph (strict)"("XScale.ScaleFit"=w298, "YScale.ScaleFit"=w298) -> ()  [unwired: 2 in, 2 out]
          n91 = property on="H(t) Graph 4" class="XYGraph (strict)"("XScale.ScaleFit"=w296, "YScale.ScaleFit"=w296) -> ()  [unwired: 2 in, 2 out]
          n92 = Build Array("Clear R(T) graph", "Clear H(T) graph", "Clear R(t) graph", "Clear T(t) graph", "Clear H(t) graph") -> (w286:bool[])
          n93 = call "Graph handler (SubVI).vi"("Data in"=w288, "Graph indices in"=w287, "Clear graph Array"=w286) -> ("Graph indices out"=w285:dbl[], "R(T) Graph"=→"R(T) Graph":cluster{dbl[], dbl[]}, "R(H) Graph"=→"R(H) Graph":cluster{dbl[], dbl[]}, "R(t) Graph"=→"R(t) Graph":cluster{dbl[], dbl[]}, "T(t) Graph 3"=→"T(t) Graph 3":cluster{dbl[], dbl[]}, "H(t) Graph 4"=→"H(t) Graph 4":cluster{dbl[], dbl[]})  [unwired: 7 in]
          n94 = node-c288() -> ()  [unwired: 1 in, 1 out]
        }
        frame #2 {
          # "Update settings"
          n95 = node-c288() -> ()  [unwired: 1 in, 1 out]
          n96 = flat-sequence {
            tunnel: w365 -> [w383]
            tunnel: w366 -> [w384]
            tunnel: w375 -> [w385]
            tunnel: w376 -> [w386]
            tunnel: w377 -> [w387]
            tunnel: [w387] -> w360
            tunnel: [w386] -> w358
            tunnel: [w385] -> w356
            tunnel: [w382] -> w354
            tunnel: [w381] -> w352
            tunnel: [w379] -> w349
            tunnel: w348 -> [w379]
            tunnel: [w378] -> w345
            tunnel: w344 -> [w378]
            tunnel: w360 -> [w431]
            tunnel: [w431] -> w359
            tunnel: w358 -> [w430]
            tunnel: [w430] -> w357
            tunnel: w356 -> [w429]
            tunnel: [w429] -> w355
            tunnel: w354 -> [w428]
            tunnel: [w428] -> w353
            tunnel: w352 -> [w427]
            tunnel: [w427] -> w351
            tunnel: [w425] -> w350
            tunnel: w349 -> [w425]
            tunnel: w345 -> [w424]
            tunnel: [w424] -> w342
            tunnel: [w435] -> w364
            tunnel: [w436] -> w363
            tunnel: [w458] -> w362
            tunnel: [w457] -> w361
            tunnel: w359 -> [w461]
            tunnel: w357 -> [w446]
            tunnel: w355 -> [w447]
            tunnel: w353 -> [w458]
            tunnel: w351 -> [w457]
            tunnel: w350 -> [w456]
            tunnel: [w456] -> w347
            tunnel: [w455] -> w343
            tunnel: w342 -> [w455]
            tunnel: [w445] -> w337
            tunnel: [w522] -> w374
            tunnel: w364 -> [w522]
            tunnel: [w514] -> w373
            tunnel: w363 -> [w514]
            tunnel: [w520] -> w368
            tunnel: [w519] -> w367
            tunnel: w362 -> [w518]
            tunnel: w361 -> [w517]
            tunnel: w347 -> [w516]
            tunnel: [w516] -> w346
            tunnel: w343 -> [w515]
            tunnel: [w515] -> w341
            frame #0 {
              n97 = event shown="[1] \"Close pins (safe)\": Value Change" {
                selector: _ -> [_ _]
                dyn-events: _ -> [_ _]
                timeout: 50 -> [_ _]
                tunnel: w384 -> [w389 w423]
                tunnel: w383 -> [w388 w422]
                tunnel: [w389 w418] -> w382
                tunnel: [w388 w417] -> w381
                event Timeout {
                  n98 = event-data() -> ()  [unwired: 1 in, 1 out]
                }
                event "Close pins (safe)": Value Change {
                  # "Close I-V pins"
                  # "Open common-ground link, then common rail"
                  n99 = event-data() -> ("Source"=w414:T5, "Type"=w415:T6)  [unwired: 1 in]
                  n100 = local read "V+"() -> (w395:i32)
                  n101 = local read "V-"() -> (w392:i32)
                  n102 = local read "I+"() -> (w400:i32)
                  n103 = local read "I-"() -> (w398:i32)
                  n104 = call "PinToChannel (SubVI).vi"("Pin"=w400, "Slot"=1) -> ("Channel"=w399:i32)  [unwired: 8 in]
                  n105 = call "PinToChannel (SubVI).vi"("Pin"=w398, "Slot"=2) -> ("Channel"=w396:i32)  [unwired: 8 in]
                  n106 = call "PinToChannel (SubVI).vi"("Pin"=w395, "Slot"=3) -> ("Channel"=w393:i32)  [unwired: 8 in]
                  n107 = call "PinToChannel (SubVI).vi"("Pin"=w392, "Slot"=4) -> ("Channel"=w390:i32)  [unwired: 8 in]
                  n108 = Create User Event(user event datatype=w415) -> (user event=w413:refnum<user-event>, error out=w416:errorcluster)  [unwired: 1 in]
                  n109 = Format Into String(format string="channel.close(\"%d;%d;%d;%d\")", w399, w396, w393, w390) -> (resulting string=w420:string)  [unwired: 2 in, 1 out]
                  n110 = VISA Write(VISA resource name=w423, write buffer=w420, error in (no error)=w422) -> (VISA resource name out=w411:refnum<visa-resource-name>, error out=w410:errorcluster)  [unwired: 1 out]
                  n111 = Generate User Event(user event=w413, event data cluster=w414, error in=w416) -> ()  [unwired: 1 in, 2 out]
                  n112 = Add(x=w399, y=400) -> (x+y=w405:i32)
                  n113 = Add(x=w396, y=300) -> (x+y=w404:i32)
                  n114 = Add(x=w393, y=200) -> (x+y=w403:i32)
                  n115 = Add(x=w390, y=100) -> (x+y=w402:i32)
                  n116 = Format Into String(format string="channel.open(\"%d;%d;%d;%d\")", w405, w404, w403, w402) -> (resulting string=w412:string)  [unwired: 2 in, 1 out]
                  n117 = VISA Write(VISA resource name=w411, write buffer=w412, error in (no error)=w410) -> (VISA resource name out=w418:refnum<visa-resource-name>, error out=w417:errorcluster)  [unwired: 1 out]
                }
              }
            }
            frame #1 {
              # "Wait 50ms for safe comms to Lakeshore"
              n118 = Wait (ms)(milliseconds to wait=50) -> ()  [unwired: 1 out]
            }
            frame #2 {
              # "Read settings with prepended command"
              # "Lakeshore settings"
              # "Updating measurement settings?"
              # "Output Lakeshore settings to indicators"
              n119 = event shown="[3] \"Lift pins (safe)\": Value Change" {
                selector: _ -> [_ _ _ _ _ _]
                dyn-events: _ -> [_ _ _ _ _ _]
                timeout: 50 -> [_ _ _ _ _ _]
                tunnel: w447 -> [_ w466 _ w486 w501 _]
                tunnel: ["" w464 "" w487 w500 w504] -> w448
                tunnel: [_ TRUE _ _ _ _] -> w459
                event Timeout {
                  n120 = event-data() -> ()  [unwired: 1 in, 1 out]
                }
                event "Update": Value Change {
                  # "Generate settings command string"
                  n121 = event-data() -> ()  [unwired: 1 in, 1 out]
                  n122 = local read "Autorange (0: Autorange off)"() -> (w471:u16)
                  n123 = local read "Excitation Range"() -> (w470:u16)
                  n124 = local read "Resistance Range"() -> (w472:u16)
                  n125 = local read "Excitation  (T: On)"() -> (w467:bool)
                  n126 = local read "Excitation Mode"() -> (w469:u16)
                  n127 = local read "Preferred Units (2: Ohms)"() -> (w474:u16)
                  n128 = Not(x=w467) -> (.not. x?=w468:bool)
                  n129 = Boolean To (0,1)(Boolean=w468) -> (0, 1=w473:i16)
                  n130 = Format Into String(format string="INTYPE %s,%d,%d,%d,%d,%d,%d;", w466, w469, w470, w471, w472, w473, w474) -> (resulting string=w464:string)  [unwired: 2 in, 1 out]
                }
                event "Grab settings": Value Change {
                  n131 = event-data() -> ()  [unwired: 1 in, 1 out]
                  n132 = local read "Preferred Units Ind"() -> (w476:u16)
                  n133 = local read "Excitation Mode Ind"() -> (w481:u16)
                  n134 = local read "Resistance Range Ind"() -> (w478:u16)
                  n135 = local read "Excitation Range Ind"() -> (w480:u16)
                  n136 = local read "Excitation  Ind"() -> (w477:bool)
                  n137 = local read "Autorange Ind"() -> (w479:u16)
                  n138 = local write "Autorange (0: Autorange off)"(w479) -> ()
                  n139 = local write "Preferred Units (2: Ohms)"(w476) -> ()
                  n140 = local write "Excitation  (T: On)"(w477) -> ()
                  n141 = local write "Resistance Range"(w478) -> ()
                  n142 = local write "Excitation Mode"(w481) -> ()
                  n143 = local write "Excitation Range"(w480) -> ()
                }
                event "Lift pins (safe)": Value Change {
                  # "Current off (shunt on)"
                  # "Generate settings command string"
                  n144 = event-data() -> ("Source"=w483:T5, "Type"=w482:T6)  [unwired: 1 in]
                  n145 = local read "Resistance Range Ind"() -> (w490:u16)
                  n146 = local read "Excitation Range Ind"() -> (w492:u16)
                  n147 = local read "Excitation Mode Ind"() -> (w493:u16)
                  n148 = local read "Autorange Ind"() -> (w491:u16)
                  n149 = local read "Preferred Units Ind"() -> (w489:u16)
                  n150 = Create User Event(user event datatype=w482) -> (user event=w484:refnum<user-event>, error out=w485:errorcluster)  [unwired: 1 in]
                  n151 = Format Into String(format string="INTYPE %s,%d,%d,%d,%d,%d,%d;", w486, w493, w492, w491, w490, 1, w489) -> (resulting string=w487:string)  [unwired: 2 in, 1 out]
                  n152 = Generate User Event(user event=w484, event data cluster=w483, error in=w485) -> ()  [unwired: 1 in, 2 out]
                }
                event "Close pins (safe)": Value Change {
                  # "Current on (shunt off)"
                  # "Generate settings command string"
                  n153 = event-data() -> ()  [unwired: 1 in, 2 out]
                  n154 = local read "Excitation Range Ind"() -> (w499:u16)
                  n155 = local read "Excitation Mode Ind"() -> (w502:u16)
                  n156 = local read "Resistance Range Ind"() -> (w497:u16)
                  n157 = local read "Autorange Ind"() -> (w498:u16)
                  n158 = local read "Preferred Units Ind"() -> (w495:u16)
                  n159 = Format Into String(format string="INTYPE %s,%d,%d,%d,%d,%d,%d;", w501, w502, w499, w498, w497, 0, w495) -> (resulting string=w500:string)  [unwired: 2 in, 1 out]
                }
                event "Update Heater Settings": Value Change {
                  # "Generate settings command string"
                  n160 = event-data() -> ()  [unwired: 1 in, 2 out]
                  n161 = Format Into String(format string="SETP %s %d;", "1", "Heater Setpoint") -> (resulting string=w504:string)  [unwired: 2 in, 1 out]
                }
              }
              n162 = call "ReadLakeshoreSettings (SubVI).vi"("Prepended command"=w448, "error in (no error)"=w446, "Channel Str"=w447, "Lakeshore port"=w461) -> ("error out"=w437:errorcluster, "Settings array out"=w445:i32[], "VISA Refnum out"=w438:refnum<visa-resource-name>)  [unwired: 3 in]
              n163 = Index Array(array=w445) -> (element #1=w454:i32, element #2=w453:i32, element #3=w452:i32, element #4=w451:i32, element #5=w450:i32, element #6=w449:i32)  [unwired: 6 in]
              n164 = To Unsigned Word Integer(number=w454) -> (unsigned 16bit integer=w444:u16)
              "Excitation Mode Ind" <- w444
              n165 = To Unsigned Word Integer(number=w453) -> (unsigned 16bit integer=w443:u16)
              "Excitation Range Ind" <- w443
              n166 = To Unsigned Word Integer(number=w451) -> (unsigned 16bit integer=w441:u16)
              "Resistance Range Ind" <- w441
              n167 = To Unsigned Word Integer(number=w452) -> (unsigned 16bit integer=w442:u16)
              "Autorange Ind" <- w442
              n168 = To Unsigned Word Integer(number=w449) -> (unsigned 16bit integer=w439:u16)
              "Preferred Units Ind" <- w439
              n169 = Equal To 0?(x=w450) -> (x = 0?=w440:bool)
              "Excitation  Ind" <- w440
              n170 = case shown="True" w459 {
                tunnel: w439 -> [_ w513]
                tunnel: w440 -> [_ w512]
                tunnel: w441 -> [_ w511]
                tunnel: w442 -> [_ w510]
                tunnel: w443 -> [_ w509]
                tunnel: w444 -> [_ w508]
                frame False {
                }
                frame True {
                  n171 = local write "Autorange (0: Autorange off)"(w510) -> ()
                  n172 = local write "Preferred Units (2: Ohms)"(w513) -> ()
                  n173 = local write "Excitation Range"(w509) -> ()
                  n174 = local write "Resistance Range"(w511) -> ()
                  n175 = local write "Excitation  (T: On)"(w512) -> ()
                  n176 = local write "Excitation Mode"(w508) -> ()
                }
              }
              n177 = call "ReadHeaterSettings.vi"("error in (no error)"=w437, "VISA Refnum in"=w438) -> ("error out"=w436:errorcluster, "Settings array out"=w434:dbl[], "VISA Refnum out"=w435:refnum<visa-resource-name>)  [unwired: 7 in]
              n178 = Index Array(array=w434) -> (element #1=w433:dbl, element #2=w432:dbl)  [unwired: 3 in, 1 out]
              n179 = local write "Heater Setpoint Ind"(w433) -> ()
              n180 = local write "Heater Output Ind"(w432) -> ()
            }
            frame #3 {
              # "Switchboard settings"
              # "Wait 50ms for safe comms to Lakeshore"
              n181 = event shown="[4] \"Lift pins (safe)\": Value Change" {
                selector: _ -> [_ _ _ _ _]
                dyn-events: _ -> [_ _ _ _ _]
                timeout: 50 -> [_ _ _ _ _]
                tunnel: [w525 w526 w538 w543 w554] -> w520
                tunnel: [w524 w529 w535 w542 w553] -> w519
                tunnel: w518 -> [w525 w531 w540 w547 w569]
                tunnel: w517 -> [w524 w530 w539 w546 w568]
                event Timeout {
                  n182 = event-data() -> ()  [unwired: 1 in, 3 out]
                }
                event "Open": Value Change {
                  # "Open channels on switchboard"
                  n183 = event-data() -> ()  [unwired: 1 in, 6 out]
                  n184 = local read "Channel Open/Close Array"() -> (w532:string)
                  n185 = Format Into String(format string="channel.open(\"%s\")", w532) -> (resulting string=w533:string)  [unwired: 2 in, 1 out]
                  n186 = VISA Write(VISA resource name=w531, write buffer=w533, error in (no error)=w530) -> (VISA resource name out=w528:refnum<visa-resource-name>, error out=w527:errorcluster)  [unwired: 1 out]
                  n187 = call <instrlib>:"ke37xx Error Query (Multiple).vi"("VISA resource name"=w528, "error in (no error)"=w527) -> ("VISA resource name out"=w526:refnum<visa-resource-name>, "error out"=w529:errorcluster)  [unwired: 10 in, 2 out]
                }
                event "Open All IV": Value Change {
                  # "Open all I-V channels on switchboard"
                  n188 = event-data() -> ()  [unwired: 1 in, 6 out]
                  n189 = VISA Write(VISA resource name=w540, write buffer="channel.open(\"1101:1414; 2101:2414\")", error in (no error)=w539) -> (VISA resource name out=w537:refnum<visa-resource-name>, error out=w536:errorcluster)  [unwired: 1 out]
                  n190 = call <instrlib>:"ke37xx Error Query (Multiple).vi"("VISA resource name"=w537, "error in (no error)"=w536) -> ("VISA resource name out"=w538:refnum<visa-resource-name>, "error out"=w535:errorcluster)  [unwired: 10 in, 2 out]
                }
                event "Close": Value Change {
                  # "Close specified channels on switchboard"
                  n191 = event-data() -> ()  [unwired: 1 in, 6 out]
                  n192 = local read "Channel Open/Close Array"() -> (w548:string)
                  n193 = Pick Line(multi-line string="channel.close(\"%s\")\nchannel.exclusiveclose(\"%s\")\nchannel.exclusiveslotclose(\"%s\")", line index=enum16{"Normal", "Exclusive", "Slot Exclusive"}."Normal" ("Mode (0: Normal)")) -> (output string=w549:string)  [unwired: 1 out]
                  n194 = Format Into String(format string=w549, w548) -> (resulting string=w551:string)  [unwired: 2 in, 1 out]
                  n195 = VISA Write(VISA resource name=w547, write buffer=w551, error in (no error)=w546) -> (VISA resource name out=w545:refnum<visa-resource-name>, error out=w544:errorcluster)  [unwired: 1 out]
                  n196 = call <instrlib>:"ke37xx Error Query (Multiple).vi"("VISA resource name"=w545, "error in (no error)"=w544) -> ("VISA resource name out"=w543:refnum<visa-resource-name>, "error out"=w542:errorcluster)  [unwired: 10 in, 2 out]
                }
                event "Lift pins (safe)": Value Change {
                  w560 = "channel.close(\"%s\")"
                  # "Open I-V pins"
                  # "Close common rail, then common-ground link"
                  n197 = event-data() -> ()  [unwired: 1 in, 1 out]
                  n198 = Format Into String(format string=w560, "1501:1512;2501:2512") -> (resulting string=w570:string)  [unwired: 2 in, 1 out]
                  n199 = VISA Write(VISA resource name=w569, write buffer=w570, error in (no error)=w568) -> (VISA resource name out=w565:refnum<visa-resource-name>, error out=w564:errorcluster)  [unwired: 1 out]
                  n200 = Format Into String(format string=w560, "1516,1616") -> (resulting string=w566:string)  [unwired: 2 in, 1 out]
                  n201 = VISA Write(VISA resource name=w565, write buffer=w566, error in (no error)=w564) -> (VISA resource name out=w563:refnum<visa-resource-name>, error out=w562:errorcluster)  [unwired: 1 out]
                  n202 = Format Into String(format string="channel.open(\"%s\")", "1101:1416; 2101:2416") -> (resulting string=w559:string)  [unwired: 2 in, 1 out]
                  n203 = VISA Write(VISA resource name=w563, write buffer=w559, error in (no error)=w562) -> (VISA resource name out=w556:refnum<visa-resource-name>, error out=w555:errorcluster)  [unwired: 1 out]
                  n204 = call <instrlib>:"ke37xx Error Query (Multiple).vi"("VISA resource name"=w556, "error in (no error)"=w555) -> ("VISA resource name out"=w554:refnum<visa-resource-name>, "error out"=w553:errorcluster)  [unwired: 10 in, 2 out]
                }
              }
              n205 = Wait (ms)(milliseconds to wait=50) -> ()  [unwired: 1 out]
              "Lakeshore Error" <- w514
            }
          }
          n206 = local read "Measurement\nperiod"() -> (w369:i64)
          n207 = Subtract(x=w339, y=0.5) -> (x-y=w338:dbl)
          n208 = node-c288(w369) -> ()  [unwired: 7 in, 1 out]
        }
      }
    }
    n209 = node-c288() -> ()  [unwired: 1 in, 1 out]
    n210 = node-c288() -> ()  [unwired: 1 in, 1 out]
  }
  n211 = node-c288(w49) -> ()  [unwired: 7 out]
